vi "Weather Parse Test.vi"() -> ()   [LabVIEW 2020, in "CDM-Config.lvlib"] (continued)
MI and Port Austin to Harbor Beach MI.\\n\\n* WHEN...The maximum winds are expected around 7 AM EST Thursday\\nwith the largest waves expected around 9 AM EST Thursday.\\n\\n* IMPACTS...Conditions will be hazardous to small craft.\",\n                \"instruction\": \"Inexperienced mariners, especially those operating smaller\\nvessels, should avoid navigating in hazardous conditions.\",\n                \"response\": \"Avoid\",\n                \"parameters\": {\n                    \"AWIPSidentifier\": [\n                        \"MWWDTX\"\n                    ],\n                    \"WMOidentifier\": [\n                        \"WHUS73 KDTX 030901\"\n                    ],\n                    \"NWSheadline\": [\n                        \"SMALL CRAFT ADVISORY REMAINS IN EFFECT UNTIL 4 PM EST THURSDAY\"\n                    ],\n                    \"BLOCKCHANNEL\": [\n                        \"EAS\",\n                        \"NWEM\",\n                        \"CMAS\"\n                    ],\n                    \"VTEC\": [\n                        \"/O.CON.KDTX.SC.Y.0091.000000T0000Z-251204T2100Z/\"\n                    ],\n                    \"eventEndingTime\": [\n                        \"2025-12-04T16:00:00-05:00\"\n                    ],\n                    \"expiredReferences\": [\n                        \"w-nws.webmaster@noaa.gov,urn:oid:2.49.0.1.840.0.2ff8cea4919408243d7957368d495bee02ffd6db.001.1,2025-12-02T03:07:00-05:00\"\n                    ]\n                },\n                \"scope\": \"Public\",\n                \"code\": \"IPAWSv1.0\",\n                \"language\": \"en-US\",\n                \"web\": \"http://www.weather.gov\",\n                \"eventCode\": {\n                    \"SAME\": [\n                        \"NWS\"\n                    ],\n                    \"NationalWeatherService\": [\n                        \"SCY\"\n                    ]\n                }\n            }\n        },\n        {\n            \"id\": \"https://api.weather.gov/alerts/urn:oid:2.49.0.1.840.0.dab1393c914b230290374bee41bf50b08330d8fe.001.1\",\n            \"type\": \"Feature\",\n            \"geometry\": null,\n            \"properties\": {\n                \"@id\": \"https://api.weather.gov/alerts/urn:oid:2.49.0.1.840.0.dab1393c914b230290374bee41bf50b08330d8fe.001.1\",\n                \"@type\": \"wx:Alert\",\n                \"id\": \"urn:oid:2.49.0.1.840.0.dab1393c914b230290374bee41bf50b08330d8fe.001.1\",\n                \"areaDesc\": \"Harbor Beach to Port Sanilac MI; Port Sanilac to Port Huron MI\",\n                \"geocode\": {\n                    \"SAME\": [\n                        \"093442\",\n                        \"093443\"\n                    ],\n                    \"UGC\": [\n                        \"LHZ442\",\n                        \"LHZ443\"\n                    ]\n                },\n                \"affectedZones\": [\n                    \"https://api.weather.gov/zones/forecast/LHZ442\",\n                    \"https://api.weather.gov/zones/forecast/LHZ443\"\n                ],\n                \"references\": [],\n                \"sent\": \"2025-12-03T04:01:00-05:00\",\n                \"effective\": \"2025-12-03T04:01:00-05:00\",\n                \"onset\": \"2025-12-03T22:00:00-05:00\",\n                \"expires\": \"2025-12-03T16:15:00-05:00\",\n                \"ends\": \"2025-12-04T16:00:00-05:00\",\n                \"status\": \"Actual\",\n                \"messageType\": \"Alert\",\n                \"category\": \"Met\",\n                \"severity\": \"Minor\",\n                \"certainty\": \"Likely\",\n                \"urgency\": \"Expected\",\n                \"event\": \"Small Craft Advisory\",\n                \"sender\": \"w-nws.webmaster@noaa.gov\",\n                \"senderName\": \"NWS Detroit/Pontiac MI\",\n                \"headline\": \"Small Craft Advisory issued December 3 at 4:01AM EST until December 4 at 4:00PM EST by NWS Detroit/Pontiac MI\",\n                \"description\": \"* WHAT...Expect sustained winds up to 23 knots from the northwest\\nwith gusts up to 30 knots. The largest significant waves will\\nbe 4 feet with a potential maximum wave height of 5 feet.\\n\\n* WHERE...Harbor Beach to Port Sanilac MI and Port Sanilac to\\nPort Huron MI.\\n\\n* WHEN...The maximum winds are expected around 6 AM EST Thursday\\nwith the largest waves expected around 9 AM EST Thursday.\\n\\n* IMPACTS...Conditions will be hazardous to small craft.\",\n                \"instruction\": \"Inexperienced mariners, especially those operating smaller\\nvessels, should avoid navigating in hazardous conditions.\",\n                \"response\": \"Avoid\",\n                \"parameters\": {\n                    \"AWIPSidentifier\": [\n                        \"MWWDTX\"\n                    ],\n                    \"WMOidentifier\": [\n                        \"WHUS73 KDTX 030901\"\n                    ],\n                    \"NWSheadline\": [\n                        \"SMALL CRAFT ADVISORY IN EFFECT FROM 10 PM THIS EVENING TO 4 PM EST THURSDAY\"\n                    ],\n                    \"BLOCKCHANNEL\": [\n                        \"EAS\",\n                        \"NWEM\",\n                        \"CMAS\"\n                    ],\n                    \"VTEC\": [\n                        \"/O.EXB.KDTX.SC.Y.0091.251204T0300Z-251204T2100Z/\"\n                    ],\n                    \"eventEndingTime\": [\n                        \"2025-12-04T16:00:00-05:00\"\n                    ]\n                },\n                \"scope\": \"Public\",\n                \"code\": \"IPAWSv1.0\",\n                \"language\": \"en-US\",\n                \"web\": \"http://www.weather.gov\",\n                \"eventCode\": {\n                    \"SAME\": [\n                        \"NWS\"\n                    ],\n                    \"NationalWeatherService\": [\n                        \"SCY\"\n                    ]\n                }\n            }\n        },\n        {\n            \"id\": \"https://api.weather.gov/alerts/urn:oid:2.49.0.1.840.0.0ce6f9fefeeb8151c750e6368d77a21669e0c8b3.001.1\",\n            \"type\": \"Feature\",\n            \"geometry\": null,\n            \"properties\": {\n                \"@id\": \"https://api.weather.gov/alerts/urn:oid:2.49.0.1.840.0.0ce6f9fefeeb8151c750e6368d77a21669e0c8b3.001.1\",\n                \"@type\": \"wx:Alert\",\n                \"id\": \"urn:oid:2.49.0.1.840.0.0ce6f9fefeeb8151c750e6368d77a21669e0c8b3.001.1\",\n                \"areaDesc\": \"Lake Mead National Recreation Area; Lake Mead National Recreation Area\",\n                \"geocode\": {\n                    \"SAME\": [\n                        \"004015\",\n                        \"032003\"\n                    ],\n                    \"UGC\": [\n                        \"AZZ036\",\n                        \"NVZ021\"\n                    ]\n                },\n                \"affectedZones\": [\n                    \"https://api.weather.gov/zones/forecast/AZZ036\",\n                    \"https://api.weather.gov/zones/forecast/NVZ021\"\n                ],\n                \"references\": [\n                    {\n                        \"@id\": \"https://api.weather.gov/alerts/urn:oid:2.49.0.1.840.0.e1ccc9c98ec3a9bf71d0b8eee838f53e2100c777.001.1\",\n                        \"identifier\": \"urn:oid:2.49.0.1.840.0.e1ccc9c98ec3a9bf71d0b8eee838f53e2100c777.001.1\",\n                        \"sender\": \"w-nws.webmaster@noaa.gov\",\n                        \"sent\": \"2025-12-02T10:39:00-08:00\"\n                    }\n                ],\n                \"sent\": \"2025-12-03T00:46:00-08:00\",\n                \"effective\": \"2025-12-03T00:46:00-08:00\",\n                \"onset\": \"2025-12-03T09:00:00-08:00\",\n                \"expires\": \"2025-12-03T18:00:00-08:00\",\n                \"ends\": \"2025-12-03T18:00:00-08:00\",\n                \"status\": \"Actual\",\n                \"messageType\": \"Update\",\n                \"category\": \"Met\",\n                \"severity\": \"Moderate\",\n                \"certainty\": \"Likely\",\n                \"urgency\": \"Expected\",\n                \"event\": \"Lake Wind Advisory\",\n                \"sender\": \"w-nws.webmaster@noaa.gov\",\n                \"senderName\": \"NWS Las Vegas NV\",\n                \"headline\": \"Lake Wind Advisory issued December 3 at 12:46AM PST until December 3 at 6:00PM PST by NWS Las Vegas NV\",\n                \"description\": \"* WHAT...North winds 15 to 25 mph with gusts up to 35 mph expected.\\nWave heights 2 to 3 feet on Lake Mohave.\\n\\n* WHERE...Lake Mead and Lake Mohave.\\n\\n* WHEN...From 9 AM PST /10 AM MST/ this morning to 6 PM PST /7 PM\\nMST/ this evening.\\n\\n* IMPACTS...Strong winds and rough waves on area lakes will create\\nhazardous conditions for small craft.\",\n                \"instruction\": \"Winds this strong can make driving difficult, especially for high\\nprofile vehicles. Use extra caution.\",\n                \"response\": \"Execute\",\n                \"parameters\": {\n                    \"AWIPSidentifier\": [\n                        \"NPWVEF\"\n                    ],\n                    \"WMOidentifier\": [\n                        \"WWUS75 KVEF 030846\"\n                    ],\n                    \"NWSheadline\": [\n                        \"LAKE WIND ADVISORY REMAINS IN EFFECT FROM 9 AM PST /10 AM MST/ THIS MORNING TO 6 PM PST /7 PM MST/ THIS EVENING\"\n                    ],\n                    \"BLOCKCHANNEL\": [\n                        \"EAS\",\n                        \"NWEM\",\n                        \"CMAS\"\n                    ],\n                    \"VTEC\": [\n                        \"/O.CON.KVEF.LW.Y.0010.251203T1700Z-251204T0200Z/\"\n                    ],\n                    \"eventEndingTime\": [\n                        \"2025-12-03T18:00:00-08:00\"\n                    ]\n                },\n                \"scope\": \"Public\",\n                \"code\": \"IPAWSv1.0\",\n                \"language\": \"en-US\",\n                \"web\": \"http://www.weather.gov\",\n                \"eventCode\": {\n                    \"SAME\": [\n                        \"NWS\"\n                    ],\n                    \"NationalWeatherService\": [\n                        \"LWY\"\n                    ]\n                }\n            }\n        },\n        {\n            \"id\": \"https://api.weather.gov/alerts/urn:oid:2.49.0.1.840.0.0594a10134f977bf8f2849286ea6b737812d75ba.001.2\",\n            \"type\": \"Feature\",\n            \"geometry\": null,\n            \"properties\": {\n                \"@id\": \"https://api.weather.gov/alerts/urn:oid:2.49.0.1.840.0.0594a10134f977bf8f2849286ea6b737812d75ba.001.2\",\n                \"@type\": \"wx:Alert\",\n                \"id\": \"urn:oid:2.49.0.1.840.0.0594a10134f977bf8f2849286ea6b737812d75ba.001.2\",\n                \"areaDesc\": \"Northern Sangre de Cristo Mountains; East Slopes Sangre de Cristo Mountains; Johnson and Bartlett Mesas Including Raton Pass\",\n                \"geocode\": {\n                    \"SAME\": [\n                        \"035007\",\n                        \"035055\",\n                        \"035033\",\n                        \"035047\",\n                        \"035059\"\n                    ],\n                    \"UGC\": [\n                        \"NMZ213\",\n                        \"NMZ215\",\n                        \"NMZ227\"\n                    ]\n                },\n                \"affectedZones\": [\n                    \"https://api.weather.gov/zones/forecast/NMZ213\",\n                    \"https://api.weather.gov/zones/forecast/NMZ215\",\n                    \"https://api.weather.gov/zones/forecast/NMZ227\"\n                ],\n                \"references\": [],\n                \"sent\": \"2025-12-03T01:43:00-07:00\",\n                \"effective\": \"2025-12-03T01:43:00-07:00\",\n                \"onset\": \"2025-12-03T12:00:00-07:00\",\n                \"expires\": \"2025-12-03T12:00:00-07:00\",\n                \"ends\": \"2025-12-04T05:00:00-07:00\",\n                \"status\": \"Actual\",\n                \"messageType\": \"Alert\",\n                \"category\": \"Met\",\n                \"severity\": \"Severe\",\n                \"certainty\": \"Likely\",\n                \"urgency\": \"Expected\",\n                \"event\": \"Winter Storm Warning\",\n                \"sender\": \"w-nws.webmaster@noaa.gov\",\n                \"senderName\": \"NWS Albuquerque NM\",\n                \"headline\": \"Winter Storm Warning issued December 3 at 1:43AM MST until December 4 at 5:00AM MST by NWS Albuquerque NM\",\n                \"description\": \"* WHAT...Heavy snow expected. Total snow accumulations between 6 and\\n12 inches, except up to 15 inches in the mountains near the\\nColorado border, and 3 to 6 inches below 7500 feet.\\n\\n* WHERE...East Slopes Sangre de Cristo Mountains, Northern Sangre de\\nCristo Mountains, and Johnson and Bartlett Mesas Including Raton\\nPass.\\n\\n* WHEN...From noon today to 5 AM MST Thursday.\\n\\n* IMPACTS...Travel could be very difficult. Tire traction will be\\nreduced. Extend the distance between your vehicle and the vehicle\\nin front of you. This includes I-25 over Raton Pass. The hazardous\\nconditions will impact commutes this evening and Thursday morning.\\n\\n* ADDITIONAL DETAILS...Snow will begin to accumulate near the\\nColorado border late this morning, then accumulating snow will\\nbecome widespread in the afternoon. The heaviest snowfall is\\nexpected this evening, when the visibility will drop below a\\nquarter mile at times.\",\n                \"instruction\": \"If you must travel, keep an extra flashlight, food, and water in\\nyour vehicle in case of an emergency. For the latest road\\nconditions, dial 511 or 1.800.432.4269, or visit http://nmroads.com.\",\n                \"response\": \"Prepare\",\n                \"parameters\": {\n                    \"AWIPSidentifier\": [\n                        \"WSWABQ\"\n                    ],\n                    \"WMOidentifier\": [\n                        \"WWUS45 KABQ 030843\"\n                    ],\n                    \"NWSheadline\": [\n                        \"WINTER STORM WARNING IN EFFECT FROM NOON TODAY TO 5 AM MST THURSDAY\"\n                    ],\n                    \"BLOCKCHANNEL\": [\n                        \"EAS\",\n                        \"NWEM\",\n                        \"CMAS\"\n                    ],\n                    \"EAS-ORG\": [\n                        \"WXR\"\n                    ],\n                    \"VTEC\": [\n                        \"/O.NEW.KABQ.WS.W.0010.251203T1900Z-251204T1200Z/\"\n                    ],\n                    \"eventEndingTime\": [\n                        \"2025-12-04T05:00:00-07:00\"\n                    ]\n                },\n                \"scope\": \"Public\",\n                \"code\": \"IPAWSv1.0\",\n                \"language\": \"en-US\",\n                \"web\": \"http://www.weather.gov\",\n                \"eventCode\": {\n                    \"SAME\": [\n                        \"WSW\"\n                    ],\n                    \"NationalWeatherService\": [\n                        \"WSW\"\n                    ]\n                }\n            }\n        },\n        {\n            \"id\": \"https://api.weather.gov/alerts/urn:oid:2.49.0.1.840.0.0594a10134f977bf8f2849286ea6b737812d75ba.005.1\",\n            \"type\": \"Feature\",\n            \"geometry\": null,\n            \"properties\": {\n                \"@id\": \"https://api.weather.gov/alerts/urn:oid:2.49.0.1.840.0.0594a10134f977bf8f2849286ea6b737812d75ba.005.1\",\n                \"@type\": \"wx:Alert\",\n                \"id\": \"urn:oid:2.49.0.1.840.0.0594a10134f977bf8f2849286ea6b737812d75ba.005.1\",\n                \"areaDesc\": \"Central Highlands\",\n                \"geocode\": {\n                    \"SAME\": [\n                        \"035047\",\n                        \"035049\",\n                        \"035057\"\n                    ],\n                    \"UGC\": [\n                        \"NMZ223\"\n                    ]\n                },\n                \"affectedZones\": [\n                    \"https://api.weather.gov/zones/forecast/NMZ223\"\n                ],\n                \"references\": [\n                    {\n                        \"@id\": \"https://api.weather.gov/alerts/urn:oid:2.49.0.1.840.0.941388ae9bb36314f84811b9b5bde722294ef589.002.1\",\n                        \"identifier\": \"urn:oid:2.49.0.1.840.0.941388ae9bb36314f84811b9b5bde722294ef589.002.1\",\n                        \"sender\": \"w-nws.webmaster@noaa.gov\",\n                        \"sent\": \"2025-12-02T18:02:00-07:00\"\n                    }\n                ],\n                \"sent\": \"2025-12-03T01:43:00-07:00\",\n                \"effective\": \"2025-12-03T01:43:00-07:00\",\n                \"onset\": \"2025-12-03T17:00:00-07:00\",\n                \"expires\": \"2025-12-03T12:00:00-07:00\",\n                \"ends\": \"2025-12-04T05:00:00-07:00\",\n                \"status\": \"Actual\",\n                \"messageType\": \"Update\",\n                \"category\": \"Met\",\n                \"severity\": \"Moderate\",\n                \"certainty\": \"Likely\",\n                \"urgency\": \"Expected\",\n                \"event\": \"Winter Weather Advisory\",\n                \"sender\": \"w-nws.webmaster@noaa.gov\",\n                \"senderName\": \"NWS Albuquerque NM\",\n                \"headline\": \"Winter Weather Advisory issued December 3 at 1:43AM MST until December 4 at 5:00AM MST by NWS Albuquerque NM\",\n                \"description\": \"* WHAT...Snow expected. Total snow accumulations between 1 and 4\\ninches.\\n\\n* WHERE...Central Highlands.\\n\\n* WHEN...From 5 PM this afternoon to 5 AM MST Thursday.\\n\\n* IMPACTS...Plan on snow packed or icy road conditions for commutes\\nthis evening and Thursday morning. This includes I-40 between\\nMoriarty and Santa Rosa, including Clines Corners.\\n\\n* ADDITIONAL DETAILS...The heaviest snowfall will occur this evening\\nwhen the visibility will drop below a half mile at times.\",\n                \"instruction\": \"Slow down and use caution while traveling. For the latest road\\nconditions, dial 511 or 1.800.432.4269, or visit http://nmroads.com.\",\n                \"response\": \"Execute\",\n                \"parameters\": {\n                    \"AWIPSidentifier\": [\n                        \"WSWABQ\"\n                    ],\n                    \"WMOidentifier\": [\n                        \"WWUS45 KABQ 030843\"\n                    ],\n                    \"NWSheadline\": [\n                        \"WINTER WEATHER ADVISORY REMAINS IN EFFECT FROM 5 PM THIS AFTERNOON TO 5 AM MST THURSDAY\"\n                    ],\n                    \"BLOCKCHANNEL\": [\n                        \"EAS\",\n                        \"NWEM\",\n                        \"CMAS\"\n                    ],\n                    \"VTEC\": [\n                        \"/O.CON.KABQ.WW.Y.0019.251204T0000Z-251204T1200Z/\"\n                    ],\n                    \"eventEndingTime\": [\n                        \"2025-12-04T05:00:00-07:00\"\n                    ],\n                    \"expiredReferences\": [\n                        \"w-nws.webmaster@noaa.gov,urn:oid:2.49.0.1.840.0.c3d145e831a7a2c0d935c1490f6242d68170c4ec.002.1,2025-12-02T09:55:00-07:00\"\n                    ]\n                },\n                \"scope\": \"Public\",\n                \"code\": \"IPAWSv1.0\",\n                \"language\": \"en-US\",\n                \"web\": \"http://www.weather.gov\",\n                \"eventCode\": {\n                    \"SAME\": [\n                        \"NWS\"\n                    ],\n                    \"NationalWeatherService\": [\n                        \"WWY\"\n                    ]\n                }\n            }\n        },\n        {\n            \"id\": \"https://api.weather.gov/alerts/urn:oid:2.49.0.1.840.0.0594a10134f977bf8f2849286ea6b737812d75ba.003.1\",\n            \"type\": \"Feature\",\n            \"geometry\": null,\n            \"properties\": {\n                \"@id\": \"https://api.weather.gov/alerts/urn:oid:2.49.0.1.840.0.0594a10134f977bf8f2849286ea6b737812d75ba.003.1\",\n                \"@type\": \"wx:Alert\",\n                \"id\": \"urn:oid:2.49.0.1.840.0.0594a10134f977bf8f2849286ea6b737812d75ba.003.1\",\n                \"areaDesc\": \"Sandia/Manzano Mountains Including Edgewood\",\n                \"geocode\": {\n                    \"SAME\": [\n                        \"035001\",\n                        \"035043\",\n                        \"035049\",\n                        \"035057\",\n                        \"035061\"\n                    ],\n                    \"UGC\": [\n                        \"NMZ221\"\n                    ]\n                },\n                \"affectedZones\": [\n                    \"https://api.weather.gov/zones/forecast/NMZ221\"\n                ],\n                \"references\": [],\n                \"sent\": \"2025-12-03T01:43:00-07:00\",\n                \"effective\": \"2025-12-03T01:43:00-07:00\",\n                \"onset\": \"2025-12-03T17:00:00-07:00\",\n                \"expires\": \"2025-12-03T12:00:00-07:00\",\n                \"ends\": \"2025-12-04T05:00:00-07:00\",\n                \"status\": \"Actual\",\n                \"messageType\": \"Alert\",\n                \"category\": \"Met\",\n                \"severity\": \"Moderate\",\n                \"certainty\": \"Likely\",\n                \"urgency\": \"Expected\",\n                \"event\": \"Winter Weather Advisory\",\n                \"sender\": \"w-nws.webmaster@noaa.gov\",\n                \"senderName\": \"NWS Albuquerque NM\",\n                \"headline\": \"Winter Weather Advisory issued December 3 at 1:43AM MST until December 4 at 5:00AM MST by NWS Albuquerque NM\",\n                \"description\": \"* WHAT...Snow expected. Total snow accumulations between 2 and 5\\ninches, with locally higher amounts on Sandia Crest.\\n\\n* WHERE...Sandia and Manzano Mountains including Edgewood.\\n\\n* WHEN...From 5 PM this afternoon to 5 AM MST Thursday.\\n\\n* IMPACTS...Plan on snow packed or icy road conditions for commutes\\nthis evening and Thursday morning. This includes I-40 through\\nTijeras Canyon.\\n\\n* ADDITIONAL DETAILS...The heaviest snow will occur this evening,\\nwhen the visibility will drop below a quarter mile at times in\\nblowing snow. East canyon wind gusts up to 35 mph during the\\nevening and through the late night hours.\",\n                \"instruction\": \"Slow down and use caution while traveling. For the latest road\\nconditions, dial 511 or 1.800.432.4269, or visit http://nmroads.com.\",\n                \"response\": \"Execute\",\n                \"parameters\": {\n                    \"AWIPSidentifier\": [\n                        \"WSWABQ\"\n                    ],\n                    \"WMOidentifier\": [\n                        \"WWUS45 KABQ 030843\"\n                    ],\n                    \"NWSheadline\": [\n                        \"WINTER WEATHER ADVISORY IN EFFECT FROM 5 PM THIS AFTERNOON TO 5 AM MST THURSDAY\"\n                    ],\n                    \"BLOCKCHANNEL\": [\n                        \"EAS\",\n                        \"NWEM\",\n                        \"CMAS\"\n                    ],\n                    \"VTEC\": [\n                        \"/O.EXA.KABQ.WW.Y.0019.251204T0000Z-251204T1200Z/\"\n                    ],\n                    \"eventEndingTime\": [\n                        \"2025-12-04T05:00:00-07:00\"\n                    ]\n                },\n                \"scope\": \"Public\",\n                \"code\": \"IPAWSv1.0\",\n                \"language\": \"en-US\",\n                \"web\": \"http://www.weather.gov\",\n                \"eventCode\": {\n                    \"SAME\": [\n                        \"NWS\"\n                    ],\n                    \"NationalWeatherService\": [\n                        \"WWY\"\n                    ]\n                }\n            }\n        },\n        {\n            \"id\": \"https://api.weather.gov/alerts/urn:oid:2.49.0.1.840.0.0594a10134f977bf8f2849286ea6b737812d75ba.002.1\",\n            \"type\": \"Feature\",\n            \"geometry\": null,\n            \"properties\": {\n                \"@id\": \"https://api.weather.gov/alerts/urn:oid:2.49.0.1.840.0.0594a10134f977bf8f2849286ea6b737812d75ba.002.1\",\n                \"@type\": \"wx:Alert\",\n                \"id\": \"urn:oid:2.49.0.1.840.0.0594a10134f977bf8f2849286ea6b737812d75ba.002.1\",\n                \"areaDesc\": \"Far Northwest Highlands; Jemez Mountains\",\n                \"geocode\": {\n                    \"SAME\": [\n                        \"035039\",\n                        \"035043\",\n                        \"035045\",\n                        \"035028\"\n                    ],\n                    \"UGC\": [\n                        \"NMZ203\",\n                        \"NMZ211\"\n                    ]\n                },\n                \"affectedZones\": [\n                    \"https://api.weather.gov/zones/forecast/NMZ203\",\n                    \"https://api.weather.gov/zones/forecast/NMZ211\"\n                ],\n                \"references\": [],\n                \"sent\": \"2025-12-03T01:43:00-07:00\",\n                \"effective\": \"2025-12-03T01:43:00-07:00\",\n                \"onset\": \"2025-12-03T12:00:00-07:00\",\n                \"expires\": \"2025-12-03T12:00:00-07:00\",\n                \"ends\": \"2025-12-04T05:00:00-07:00\",\n                \"status\": \"Actual\",\n                \"messageType\": \"Alert\",\n                \"category\": \"Met\",\n                \"severity\": \"Moderate\",\n                \"certainty\": \"Likely\",\n                \"urgency\": \"Expected\",\n                \"event\": \"Winter Weather Advisory\",\n                \"sender\": \"w-nws.webmaster@noaa.gov\",\n                \"senderName\": \"NWS Albuquerque NM\",\n                \"headline\": \"Winter Weather Advisory issued December 3 at 1:43AM MST until December 4 at 5:00AM MST by NWS Albuquerque NM\",\n                \"description\": \"* WHAT...Snow expected. Total snow accumulations between 1 and 3\\ninches, except 3 to 6 inches above 7500 feet.  Locally higher\\namounts near 8 inches along the east slopes of the Jemez Mountains.\\n\\n* WHERE...Far Northwest Highlands and Jemez Mountains.\\n\\n* WHEN...From noon today to 5 AM MST Thursday.\\n\\n* IMPACTS...Plan on snow packed or icy road conditions. The\\nhazardous conditions will impact commutes this evening and\\nThursday morning.\\n\\n* ADDITIONAL DETAILS...Snow will begin to accumulate near the\\nColorado border late this morning, then accumulating snow will\\nspread to the Jemez Mountains as well during the afternoon. The\\nheaviest snowfall will occur Wednesday evening in most places,\\nwhen the visibility will drop below a half mile at times.\",\n                \"instruction\": \"Slow down and use caution while traveling. For the latest road\\nconditions, dial 511 or 1.800.432.4269, or visit http://nmroads.com.\",\n                \"response\": \"Execute\",\n                \"parameters\": {\n                    \"AWIPSidentifier\": [\n                        \"WSWABQ\"\n                    ],\n                    \"WMOidentifier\": [\n                        \"WWUS45 KABQ 030843\"\n                    ],\n                    \"NWSheadline\": [\n                        \"WINTER WEATHER ADVISORY IN EFFECT FROM NOON TODAY TO 5 AM MST THURSDAY\"\n                    ],\n                    \"BLOCKCHANNEL\": [\n                        \"EAS\",\n                        \"NWEM\",\n                        \"CMAS\"\n                    ],\n                    \"VTEC\": [\n                        \"/O.EXA.KABQ.WW.Y.0019.251203T1900Z-251204T1200Z/\"\n                    ],\n                    \"eventEndingTime\": [\n                        \"2025-12-04T05:00:00-07:00\"\n                    ]\n                },\n                \"scope\": \"Public\",\n                \"code\": \"IPAWSv1.0\",\n                \"language\": \"en-US\",\n                \"web\": \"http://www.weather.gov\",\n                \"eventCode\": {\n                    \"SAME\": [\n                        \"NWS\"\n                    ],\n                    \"NationalWeatherService\": [\n                        \"WWY\"\n                    ]\n                }\n            }\n        },\n        {\n            \"id\": \"https://api.weather.gov/alerts/urn:oid:2.49.0.1.840.0.0594a10134f977bf8f2849286ea6b737812d75ba.004.1\",\n            \"type\": \"Feature\",\n            \"geometry\": null,\n            \"properties\": {\n                \"@id\": \"https://api.weather.gov/alerts/urn:oid:2.49.0.1.840.0.0594a10134f977bf8f2849286ea6b737812d75ba.004.1\",\n                \"@type\": \"wx:Alert\",\n                \"id\": \"urn:oid:2.49.0.1.840.0.0594a10134f977bf8f2849286ea6b737812d75ba.004.1\",\n                \"areaDesc\": \"Tusas Mountains Including Chama; Glorieta Mesa Including Glorieta Pass; Southern Sangre de Cristo Mountains; Upper Rio Grande Valley; Far Northeast Highlands; Northeast Highlands\",\n                \"geocode\": {\n                    \"SAME\": [\n                        \"035039\",\n                        \"035055\",\n                        \"035047\",\n                        \"035049\",\n                        \"035007\",\n                        \"035033\"\n                    ],\n                    \"UGC\": [\n                        \"NMZ210\",\n                        \"NMZ212\",\n                        \"NMZ214\",\n                        \"NMZ216\",\n                        \"NMZ228\",\n                        \"NMZ229\"\n                    ]\n                },\n                \"affectedZones\": [\n                    \"https://api.weather.gov/zones/forecast/NMZ210\",\n                    \"https://api.weather.gov/zones/forecast/NMZ212\",\n                    \"https://api.weather.gov/zones/forecast/NMZ214\",\n                    \"https://api.weather.gov/zones/forecast/NMZ216\",\n                    \"https://api.weather.gov/zones/forecast/NMZ228\",\n                    \"https://api.weather.gov/zones/forecast/NMZ229\"\n                ],\n                \"references\": [\n                    {\n                        \"@id\": \"https://api.weather.gov/alerts/urn:oid:2.49.0.1.840.0.941388ae9bb36314f84811b9b5bde722294ef589.001.1\",\n                        \"identifier\": \"urn:oid:2.49.0.1.840.0.941388ae9bb36314f84811b9b5bde722294ef589.001.1\",\n                        \"sender\": \"w-nws.webmaster@noaa.gov\",\n                        \"sent\": \"2025-12-02T18:02:00-07:00\"\n                    }\n                ],\n                \"sent\": \"2025-12-03T01:43:00-07:00\",\n                \"effective\": \"2025-12-03T01:43:00-07:00\",\n                \"onset\": \"2025-12-03T12:00:00-07:00\",\n                \"expires\": \"2025-12-03T12:00:00-07:00\",\n                \"ends\": \"2025-12-04T05:00:00-07:00\",\n                \"status\": \"Actual\",\n                \"messageType\": \"Update\",\n                \"category\": \"Met\",\n                \"severity\": \"Moderate\",\n                \"certainty\": \"Likely\",\n                \"urgency\": \"Expected\",\n                \"event\": \"Winter Weather Advisory\",\n                \"sender\": \"w-nws.webmaster@noaa.gov\",\n                \"senderName\": \"NWS Albuquerque NM\",\n                \"headline\": \"Winter Weather Advisory issued December 3 at 1:43AM MST until December 4 at 5:00AM MST by NWS Albuquerque NM\",\n                \"description\": \"* WHAT...Snow expected. Total snow accumulations between 1 and 4\\ninches below 7500 feet, and between 4 and 8 inches above 7500\\nfeet. Locally up to 10 inches on the highest peaks of the Sangre\\nde Cristo Mountains.\\n\\n* WHERE...Glorieta Mesa Including Glorieta Pass, Southern Sangre de\\nCristo Mountains, Tusas Mountains Including Chama, Upper Rio\\nGrande Valley, Far Northeast Highlands, and Northeast Highlands.\\n\\n* WHEN...From noon today to 5 AM MST Thursday.\\n\\n* IMPACTS...Travel could be very difficult. Tire traction will be\\nreduced. Extend the distance between your vehicle and the vehicle\\nin front of you. This includes I-25 over Glorieta Pass. The\\nhazardous conditions will impact commutes this evening and\\nThursday morning.\\n\\n* ADDITIONAL DETAILS...Snow will begin to accumulate near the\\nColorado border this morning, then spread further south this\\nafternoon.  The heaviest snowfall in most locations will occur\\nthis evening when the visibility will drop below a half mile at\\ntimes.\",\n                \"instruction\": \"Slow down and use caution while traveling. For the latest road\\nconditions, dial 511 or 1.800.432.4269, or visit http://nmroads.com.\",\n                \"response\": \"Execute\",\n                \"parameters\": {\n                    \"AWIPSidentifier\": [\n                        \"WSWABQ\"\n                    ],\n                    \"WMOidentifier\": [\n                        \"WWUS45 KABQ 030843\"\n                    ],\n                    \"NWSheadline\": [\n                        \"WINTER WEATHER ADVISORY REMAINS IN EFFECT FROM NOON TODAY TO 5 AM MST THURSDAY\"\n                    ],\n                    \"BLOCKCHANNEL\": [\n                        \"EAS\",\n                        \"NWEM\",\n                        \"CMAS\"\n                    ],\n                    \"VTEC\": [\n                        \"/O.CON.KABQ.WW.Y.0019.251203T1900Z-251204T1200Z/\"\n                    ],\n                    \"eventEndingTime\": [\n                        \"2025-12-04T05:00:00-07:00\"\n                    ],\n                    \"expiredReferences\": [\n                        \"w-nws.webmaster@noaa.gov,urn:oid:2.49.0.1.840.0.c3d145e831a7a2c0d935c1490f6242d68170c4ec.003.1,2025-12-02T09:55:00-07:00 w-nws.webmaster@noaa.gov,urn:oid:2.49.0.1.840.0.c3d145e831a7a2c0d935c1490f6242d68170c4ec.001.1,2025-12-02T09:55:00-07:00 w-nws.webmaster@noaa.gov,urn:oid:2.49.0.1.840.0.0ace8003fd2e1ec30d59fe0304cfb7a59138cfec.001.1,2025-12-02T02:40:00-07:00\"\n                    ]\n                },\n                \"scope\": \"Public\",\n                \"code\": \"IPAWSv1.0\",\n                \"language\": \"en-US\",\n                \"web\": \"http://www.weather.gov\",\n                \"eventCode\": {\n                    \"SAME\": [\n                        \"NWS\"\n                    ],\n                    \"NationalWeatherService\": [\n                        \"WWY\"\n                    ]\n                }\n            }\n        },\n        {\n            \"id\": \"https://api.weather.gov/alerts/urn:oid:2.49.0.1.840.0.810f735991b3c019dc43a3db04dbca83dd500741.001.1\",\n            \"type\": \"Feature\",\n            \"geometry\": null,\n            \"properties\": {\n                \"@id\": \"https://api.weather.gov/alerts/urn:oid:2.49.0.1.840.0.810f735991b3c019dc43a3db04dbca83dd500741.001.1\",\n                \"@type\": \"wx:Alert\",\n                \"id\": \"urn:oid:2.49.0.1.840.0.810f735991b3c019dc43a3db04dbca83dd500741.001.1\",\n                \"areaDesc\": \"Greater Lake Tahoe Area; Greater Lake Tahoe Area\",\n                \"geocode\": {\n                    \"SAME\": [\n                        \"006003\",\n                        \"006017\",\n                        \"006057\",\n                        \"006061\",\n                        \"032005\",\n                        \"032031\",\n                        \"032510\"\n                    ],\n                    \"UGC\": [\n                        \"CAZ072\",\n                        \"NVZ002\"\n                    ]\n                },\n                \"affectedZones\": [\n                    \"https://api.weather.gov/zones/forecast/CAZ072\",\n                    \"https://api.weather.gov/zones/forecast/NVZ002\"\n                ],\n                \"references\": [],\n                \"sent\": \"2025-12-03T00:34:00-08:00\",\n                \"effective\": \"2025-12-03T00:34:00-08:00\",\n                \"onset\": \"2025-12-03T00:34:00-08:00\",\n                \"expires\": \"2025-12-03T10:00:00-08:00\",\n                \"ends\": \"2025-12-03T10:00:00-08:00\",\n                \"status\": \"Actual\",\n                \"messageType\": \"Alert\",\n                \"category\": \"Met\",\n                \"severity\": \"Moderate\",\n                \"certainty\": \"Likely\",\n                \"urgency\": \"Expected\",\n                \"event\": \"Lake Wind Advisory\",\n                \"sender\": \"w-nws.webmaster@noaa.gov\",\n                \"senderName\": \"NWS Reno NV\",\n                \"headline\": \"Lake Wind Advisory issued December 3 at 12:34AM PST until December 3 at 10:00AM PST by NWS Reno NV\",\n                \"description\": \"* WHAT...East winds 15 to 20 mph with gusts up to 35 mph and waves 1\\nto 3 feet for Lake Tahoe.\\n\\n* WHERE...Greater Lake Tahoe Area.\\n\\n* WHEN...Until 10 AM PST this morning.\\n\\n* IMPACTS...Small boats, kayaks and paddle boards will be prone to\\ncapsizing and should remain off lake waters until conditions\\nimprove.\\n\\n* ADDITIONAL DETAILS...The strongest winds and highest waves will\\noccur over the southwest portion of Lake Tahoe.\",\n                \"instruction\": \"Check lake conditions before heading out and be prepared for a\\nsudden increase in winds and wave heights. Consider postponing\\nboating activities on the lake until a day with less wind.\",\n                \"response\": \"Execute\",\n                \"parameters\": {\n                    \"AWIPSidentifier\": [\n                        \"NPWREV\"\n                    ],\n                    \"WMOidentifier\": [\n                        \"WWUS75 KREV 030834\"\n                    ],\n                    \"NWSheadline\": [\n                        \"LAKE WIND ADVISORY IN EFFECT UNTIL 10 AM PST THIS MORNING FOR LAKE TAHOE\"\n                    ],\n                    \"BLOCKCHANNEL\": [\n                        \"EAS\",\n                        \"NWEM\",\n                        \"CMAS\"\n                    ],\n                    \"VTEC\": [\n                        \"/O.NEW.KREV.LW.Y.0041.251203T0834Z-251203T1800Z/\"\n                    ],\n                    \"eventEndingTime\": [\n                        \"2025-12-03T10:00:00-08:00\"\n                    ]\n                },\n                \"scope\": \"Public\",\n                \"code\": \"IPAWSv1.0\",\n                \"language\": \"en-US\",\n                \"web\": \"http://www.weather.gov\",\n                \"eventCode\": {\n                    \"SAME\": [\n                        \"NWS\"\n                    ],\n                    \"NationalWeatherService\": [\n                        \"LWY\"\n                    ]\n                }\n            }\n        },\n        {\n            \"id\": \"https://api.weather.gov/alerts/urn:oid:2.49.0.1.840.0.e553a78eb2e76c08ee00c537b77b6bdc9b00773a.005.1\",\n            \"type\": \"Feature\",\n            \"geometry\": null,\n            \"properties\": {\n                \"@id\": \"https://api.weather.gov/alerts/urn:oid:2.49.0.1.840.0.e553a78eb2e76c08ee00c537b77b6bdc9b00773a.005.1\",\n                \"@type\": \"wx:Alert\",\n                \"id\": \"urn:oid:2.49.0.1.840.0.e553a78eb2e76c08ee00c537b77b6bdc9b00773a.005.1\",\n                \"areaDesc\": \"Mexico Bay NY to the St. Lawrence River\",\n                \"geocode\": {\n                    \"SAME\": [\n                        \"097045\"\n                    ],\n                    \"UGC\": [\n                        \"LOZ045\"\n                    ]\n                },\n                \"affectedZones\": [\n                    \"https://api.weather.gov/zones/forecast/LOZ045\"\n                ],\n                \"references\": [\n                    {\n                        \"@id\": \"https://api.weather.gov/alerts/urn:oid:2.49.0.1.840.0.f324634d91b7df287210abe8d836b370d8caadcc.005.1\",\n                        \"identifier\": \"urn:oid:2.49.0.1.840.0.f324634d91b7df287210abe8d836b370d8caadcc.005.1\",\n                        \"sender\": \"w-nws.webmaster@noaa.gov\",\n                        \"sent\": \"2025-12-02T15:44:00-05:00\"\n                    }\n                ],\n                \"sent\": \"2025-12-03T03:34:00-05:00\",\n                \"effective\": \"2025-12-03T03:34:00-05:00\",\n                \"onset\": \"2025-12-03T13:00:00-05:00\",\n                \"expires\": \"2025-12-03T13:00:00-05:00\",\n                \"ends\": \"2025-12-05T01:00:00-05:00\",\n                \"status\": \"Actual\",\n                \"messageType\": \"Update\",\n                \"category\": \"Met\",\n                \"severity\": \"Minor\",\n                \"certainty\": \"Likely\",\n                \"urgency\": \"Expected\",\n                \"event\": \"Small Craft Advisory\",\n                \"sender\": \"w-nws.webmaster@noaa.gov\",\n                \"senderName\": \"NWS Buffalo NY\",\n                \"headline\": \"Small Craft Advisory issued December 3 at 3:34AM EST until December 5 at 1:00AM EST by NWS Buffalo NY\",\n                \"description\": \"* WHAT...Southwest to west winds to 30 knots and waves 8 to 11\\nfeet expected.\\n\\n* WHERE...The nearshore waters of Lake Ontario from Mexico Bay\\nto the Saint Lawrence River.\\n\\n* WHEN...From 1 PM this afternoon to 1 AM EST Friday.\\n\\n* IMPACTS...Winds and/or waves will cause hazardous conditions\\nthat could capsize or damage small craft.\",\n                \"instruction\": \"Inexperienced mariners, especially those operating smaller\\nvessels, should avoid navigating in hazardous conditions.\",\n                \"response\": \"Avoid\",\n                \"parameters\": {\n                    \"AWIPSidentifier\": [\n                        \"MWWBUF\"\n                    ],\n                    \"WMOidentifier\": [\n                        \"WHUS71 KBUF 030834\"\n                    ],\n                    \"NWSheadline\": [\n                        \"SMALL CRAFT ADVISORY REMAINS IN EFFECT FROM 1 PM THIS AFTERNOON TO 1 AM EST FRIDAY\"\n                    ],\n                    \"BLOCKCHANNEL\": [\n                        \"EAS\",\n                        \"NWEM\",\n                        \"CMAS\"\n                    ],\n                    \"VTEC\": [\n                        \"/O.CON.KBUF.SC.Y.0098.251203T1800Z-251205T0600Z/\"\n                    ],\n                    \"eventEndingTime\": [\n                        \"2025-12-05T01:00:00-05:00\"\n                    ]\n                },\n                \"scope\": \"Public\",\n                \"code\": \"IPAWSv1.0\",\n                \"language\": \"en-US\",\n                \"web\": \"http://www.weather.gov\",\n                \"eventCode\": {\n                    \"SAME\": [\n                        \"NWS\"\n                    ],\n                    \"NationalWeatherService\": [\n                        \"SCY\"\n                    ]\n                }\n            }\n        },\n        {\n            \"id\": \"https://api.weather.gov/alerts/urn:oid:2.49.0.1.840.0.e553a78eb2e76c08ee00c537b77b6bdc9b00773a.004.1\",\n            \"type\": \"Feature\",\n            \"geometry\": null,\n            \"properties\": {\n                \"@id\": \"https://api.weather.gov/alerts/urn:oid:2.49.0.1.840.0.e553a78eb2e76c08ee00c537b77b6bdc9b00773a.004.1\",\n                \"@type\": \"wx:Alert\",\n                \"id\": \"urn:oid:2.49.0.1.840.0.e553a78eb2e76c08ee00c537b77b6bdc9b00773a.004.1\",\n                \"areaDesc\": \"Hamlin Beach to Sodus Bay NY; Sodus Bay to Mexico Bay NY\",\n                \"geocode\": {\n                    \"SAME\": [\n                        \"097043\",\n                        \"097044\"\n                    ],\n                    \"UGC\": [\n                        \"LOZ043\",\n                        \"LOZ044\"\n                    ]\n                },\n                \"affectedZones\": [\n                    \"https://api.weather.gov/zones/forecast/LOZ043\",\n                    \"https://api.weather.gov/zones/forecast/LOZ044\"\n                ],\n                \"references\": [\n                    {\n                        \"@id\": \"https://api.weather.gov/alerts/urn:oid:2.49.0.1.840.0.f324634d91b7df287210abe8d836b370d8caadcc.004.1\",\n                        \"identifier\": \"urn:oid:2.49.0.1.840.0.f324634d91b7df287210abe8d836b370d8caadcc.004.1\",\n                        \"sender\": \"w-nws.webmaster@noaa.gov\",\n                        \"sent\": \"2025-12-02T15:44:00-05:00\"\n                    }\n                ],\n                \"sent\": \"2025-12-03T03:34:00-05:00\",\n                \"effective\": \"2025-12-03T03:34:00-05:00\",\n                \"onset\": \"2025-12-03T19:00:00-05:00\",\n                \"expires\": \"2025-12-03T13:00:00-05:00\",\n                \"ends\": \"2025-12-05T01:00:00-05:00\",\n                \"status\": \"Actual\",\n                \"messageType\": \"Update\",\n                \"category\": \"Met\",\n                \"severity\": \"Minor\",\n                \"certainty\": \"Likely\",\n                \"urgency\": \"Expected\",\n                \"event\": \"Small Craft Advisory\",\n                \"sender\": \"w-nws.webmaster@noaa.gov\",\n                \"senderName\": \"NWS Buffalo NY\",\n                \"headline\": \"Small Craft Advisory issued December 3 at 3:34AM EST until December 5 at 1:00AM EST by NWS Buffalo NY\",\n                \"description\": \"* WHAT...Southwest to west winds to 30 knots and waves 10 to 13\\nfeet expected.\\n\\n* WHERE...The nearshore waters of Lake Ontario from Hamlin Beach\\nto Mexico Bay.\\n\\n* WHEN...From 7 PM this evening to 1 AM EST Friday.\\n\\n* IMPACTS...Winds and/or waves will cause hazardous conditions\\nthat could capsize or damage small craft.\",\n                \"instruction\": \"Inexperienced mariners, especially those operating smaller\\nvessels, should avoid navigating in hazardous conditions.\",\n                \"response\": \"Avoid\",\n                \"parameters\": {\n                    \"AWIPSidentifier\": [\n                        \"MWWBUF\"\n                    ],\n                    \"WMOidentifier\": [\n                        \"WHUS71 KBUF 030834\"\n                    ],\n                    \"NWSheadline\": [\n                        \"SMALL CRAFT ADVISORY REMAINS IN EFFECT FROM 7 PM THIS EVENING TO 1 AM EST FRIDAY\"\n                    ],\n                    \"BLOCKCHANNEL\": [\n                        \"EAS\",\n                        \"NWEM\",\n                        \"CMAS\"\n                    ],\n                    \"VTEC\": [\n                        \"/O.CON.KBUF.SC.Y.0098.251204T0000Z-251205T0600Z/\"\n                    ],\n                    \"eventEndingTime\": [\n                        \"2025-12-05T01:00:00-05:00\"\n                    ]\n                },\n                \"scope\": \"Public\",\n                \"code\": \"IPAWSv1.0\",\n                \"language\": \"en-US\",\n                \"web\": \"http://www.weather.gov\",\n                \"eventCode\": {\n                    \"SAME\": [\n                        \"NWS\"\n                    ],\n                    \"NationalWeatherService\": [\n                        \"SCY\"\n                    ]\n                }\n            }\n        },\n        {\n            \"id\": \"https://api.weather.gov/alerts/urn:oid:2.49.0.1.840.0.e553a78eb2e76c08ee00c537b77b6bdc9b00773a.002.1\",\n            \"type\": \"Feature\",\n            \"geometry\": null,\n            \"properties\": {\n                \"@id\": \"https://api.weather.gov/alerts/urn:oid:2.49.0.1.840.0.e553a78eb2e76c08ee00c537b77b6bdc9b00773a.002.1\",\n                \"@type\": \"wx:Alert\",\n                \"id\": \"urn:oid:2.49.0.1.840.0.e553a78eb2e76c08ee00c537b77b6bdc9b00773a.002.1\",\n                \"areaDesc\": \"Upper Niagara River and Buffalo Harbor; Lower Niagara River\",\n                \"geocode\": {\n                    \"SAME\": [\n                        \"096020\",\n                        \"097030\"\n                    ],\n                    \"UGC\": [\n                        \"LEZ020\",\n                        \"LOZ030\"\n                    ]\n                },\n                \"affectedZones\": [\n                    \"https://api.weather.gov/zones/forecast/LEZ020\",\n                    \"https://api.weather.gov/zones/forecast/LOZ030\"\n                ],\n                \"references\": [\n                    {\n                        \"@id\": \"https://api.weather.gov/alerts/urn:oid:2.49.0.1.840.0.f324634d91b7df287210abe8d836b370d8caadcc.002.1\",\n                        \"identifier\": \"urn:oid:2.49.0.1.840.0.f324634d91b7df287210abe8d836b370d8caadcc.002.1\",\n                        \"sender\": \"w-nws.webmaster@noaa.gov\",\n                        \"sent\": \"2025-12-02T15:44:00-05:00\"\n                    }\n                ],\n                \"sent\": \"2025-12-03T03:34:00-05:00\",\n                \"effective\": \"2025-12-03T03:34:00-05:00\",\n                \"onset\": \"2025-12-03T11:00:00-05:00\",\n                \"expires\": \"2025-12-03T13:00:00-05:00\",\n                \"ends\": \"2025-12-04T19:00:00-05:00\",\n                \"status\": \"Actual\",\n                \"messageType\": \"Update\",\n                \"category\": \"Met\",\n                \"severity\": \"Minor\",\n                \"certainty\": \"Likely\",\n                \"urgency\": \"Expected\",\n                \"event\": \"Small Craft Advisory\",\n                \"sender\": \"w-nws.webmaster@noaa.gov\",\n                \"senderName\": \"NWS Buffalo NY\",\n                \"headline\": \"Small Craft Advisory issued December 3 at 3:34AM EST until December 4 at 7:00PM EST by NWS Buffalo NY\",\n                \"description\": \"* WHAT...Southwest to west winds 15 to 20 knots expected.\\n\\n* WHERE...The Niagara River and Buffalo Harbor.\\n\\n* WHEN...From 11 AM this morning to 7 PM EST Thursday.\\n\\n* IMPACTS...Winds and/or waves will cause hazardous conditions\\nthat could capsize or damage small craft.\",\n                \"instruction\": \"Inexperienced mariners, especially those operating smaller\\nvessels, should avoid navigating in hazardous conditions.\",\n                \"response\": \"Avoid\",\n                \"parameters\": {\n                    \"AWIPSidentifier\": [\n                        \"MWWBUF\"\n                    ],\n                    \"WMOidentifier\": [\n                        \"WHUS71 KBUF 030834\"\n                    ],\n                    \"NWSheadline\": [\n                        \"SMALL CRAFT ADVISORY REMAINS IN EFFECT FROM 11 AM THIS MORNING TO 7 PM EST THURSDAY\"\n                    ],\n                    \"BLOCKCHANNEL\": [\n                        \"EAS\",\n                        \"NWEM\",\n                        \"CMAS\"\n                    ],\n                    \"VTEC\": [\n                        \"/O.CON.KBUF.SC.Y.0098.251203T1600Z-251205T0000Z/\"\n                    ],\n                    \"eventEndingTime\": [\n                        \"2025-12-04T19:00:00-05:00\"\n                    ]\n                },\n                \"scope\": \"Public\",\n                \"code\": \"IPAWSv1.0\",\n                \"language\": \"en-US\",\n                \"web\": \"http://www.weather.gov\",\n                \"eventCode\": {\n                    \"SAME\": [\n                        \"NWS\"\n                    ],\n                    \"NationalWeatherService\": [\n                        \"SCY\"\n                    ]\n                }\n            }\n        },\n        {\n            \"id\": \"https://api.weather.gov/alerts/urn:oid:2.49.0.1.840.0.e553a78eb2e76c08ee00c537b77b6bdc9b00773a.003.1\",\n            \"type\": \"Feature\",\n            \"geometry\": null,\n            \"properties\": {\n                \"@id\": \"https://api.weather.gov/alerts/urn:oid:2.49.0.1.840.0.e553a78eb2e76c08ee00c537b77b6bdc9b00773a.003.1\",\n                \"@type\": \"wx:Alert\",\n                \"id\": \"urn:oid:2.49.0.1.840.0.e553a78eb2e76c08ee00c537b77b6bdc9b00773a.003.1\",\n                \"areaDesc\": \"Niagara River to Hamlin Beach NY\",\n                \"geocode\": {\n                    \"SAME\": [\n                        \"097042\"\n                    ],\n                    \"UGC\": [\n                        \"LOZ042\"\n                    ]\n                },\n                \"affectedZones\": [\n                    \"https://api.weather.gov/zones/forecast/LOZ042\"\n                ],\n                \"references\": [\n                    {\n                        \"@id\": \"https://api.weather.gov/alerts/urn:oid:2.49.0.1.840.0.f324634d91b7df287210abe8d836b370d8caadcc.003.1\",\n                        \"identifier\": \"urn:oid:2.49.0.1.840.0.f324634d91b7df287210abe8d836b370d8caadcc.003.1\",\n                        \"sender\": \"w-nws.webmaster@noaa.gov\",\n                        \"sent\": \"2025-12-02T15:44:00-05:00\"\n                    }\n                ],\n                \"sent\": \"2025-12-03T03:34:00-05:00\",\n                \"effective\": \"2025-12-03T03:34:00-05:00\",\n                \"onset\": \"2025-12-03T11:00:00-05:00\",\n                \"expires\": \"2025-12-03T13:00:00-05:00\",\n                \"ends\": \"2025-12-04T22:00:00-05:00\",\n                \"status\": \"Actual\",\n                \"messageType\": \"Update\",\n                \"category\": \"Met\",\n                \"severity\": \"Minor\",\n                \"certainty\": \"Likely\",\n                \"urgency\": \"Expected\",\n                \"event\": \"Small Craft Advisory\",\n                \"sender\": \"w-nws.webmaster@noaa.gov\",\n                \"senderName\": \"NWS Buffalo NY\",\n                \"headline\": \"Small Craft Advisory issued December 3 at 3:34AM EST until December 4 at 10:00PM EST by NWS Buffalo NY\",\n                \"description\": \"* WHAT...Southwest to west winds to 30 knots and waves 7 to 10\\nfeet expected.\\n\\n* WHERE...The nearshore waters of Lake Ontario from the Niagara\\nRiver to Hamlin Beach.\\n\\n* WHEN...From 11 AM this morning to 10 PM EST Thursday.\\n\\n* IMPACTS...Winds and/or waves will cause hazardous conditions\\nthat could capsize or damage small craft.\",\n                \"instruction\": \"Inexperienced mariners, especially those operating smaller\\nvessels, should avoid navigating in hazardous conditions.\",\n                \"response\": \"Avoid\",\n                \"parameters\": {\n                    \"AWIPSidentifier\": [\n                        \"MWWBUF\"\n                    ],\n                    \"WMOidentifier\": [\n                        \"WHUS71 KBUF 030834\"\n                    ],\n                    \"NWSheadline\": [\n                        \"SMALL CRAFT ADVISORY REMAINS IN EFFECT FROM 11 AM THIS MORNING TO 10 PM EST THURSDAY\"\n                    ],\n                    \"BLOCKCHANNEL\": [\n                        \"EAS\",\n                        \"NWEM\",\n                        \"CMAS\"\n                    ],\n                    \"VTEC\": [\n                        \"/O.CON.KBUF.SC.Y.0098.251203T1600Z-251205T0300Z/\"\n                    ],\n                    \"eventEndingTime\": [\n                        \"2025-12-04T22:00:00-05:00\"\n                    ]\n                },\n                \"scope\": \"Public\",\n                \"code\": \"IPAWSv1.0\",\n                \"language\": \"en-US\",\n                \"web\": \"http://www.weather.gov\",\n                \"eventCode\": {\n                    \"SAME\": [\n                        \"NWS\"\n                    ],\n                    \"NationalWeatherService\": [\n                        \"SCY\"\n                    ]\n                }\n            }\n        },\n        {\n            \"id\": \"https://api.weather.gov/alerts/urn:oid:2.49.0.1.840.0.e553a78eb2e76c08ee00c537b77b6bdc9b00773a.001.1\",\n            \"type\": \"Feature\",\n            \"geometry\": null,\n            \"properties\": {\n                \"@id\": \"https://api.weather.gov/alerts/urn:oid:2.49.0.1.840.0.e553a78eb2e76c08ee00c537b77b6bdc9b00773a.001.1\",\n                \"@type\": \"wx:Alert\",\n                \"id\": \"urn:oid:2.49.0.1.840.0.e553a78eb2e76c08ee00c537b77b6bdc9b00773a.001.1\",\n                \"areaDesc\": \"Ripley to Dunkirk NY; Dunkirk to Buffalo NY\",\n                \"geocode\": {\n                    \"SAME\": [\n                        \"096040\",\n                        \"096041\"\n                    ],\n                    \"UGC\": [\n                        \"LEZ040\",\n                        \"LEZ041\"\n                    ]\n                },\n                \"affectedZones\": [\n                    \"https://api.weather.gov/zones/forecast/LEZ040\",\n                    \"https://api.weather.gov/zones/forecast/LEZ041\"\n                ],\n                \"references\": [\n                    {\n                        \"@id\": \"https://api.weather.gov/alerts/urn:oid:2.49.0.1.840.0.f324634d91b7df287210abe8d836b370d8caadcc.001.1\",\n                        \"identifier\": \"urn:oid:2.49.0.1.840.0.f324634d91b7df287210abe8d836b370d8caadcc.001.1\",\n                        \"sender\": \"w-nws.webmaster@noaa.gov\",\n                        \"sent\": \"2025-12-02T15:44:00-05:00\"\n                    }\n                ],\n                \"sent\": \"2025-12-03T03:34:00-05:00\",\n                \"effective\": \"2025-12-03T03:34:00-05:00\",\n                \"onset\": \"2025-12-03T07:00:00-05:00\",\n                \"expires\": \"2025-12-03T13:00:00-05:00\",\n                \"ends\": \"2025-12-04T22:00:00-05:00\",\n                \"status\": \"Actual\",\n                \"messageType\": \"Update\",\n                \"category\": \"Met\",\n                \"severity\": \"Minor\",\n                \"certainty\": \"Likely\",\n                \"urgency\": \"Expected\",\n                \"event\": \"Small Craft Advisory\",\n                \"sender\": \"w-nws.webmaster@noaa.gov\",\n                \"senderName\": \"NWS Buffalo NY\",\n                \"headline\": \"Small Craft Advisory issued December 3 at 3:34AM EST until December 4 at 10:00PM EST by NWS Buffalo NY\",\n                \"description\": \"* WHAT...Southwest to west winds to 30 knots and waves 7 to 10\\nfeet expected.\\n\\n* WHERE...The nearshore waters of Lake Erie from Ripley to\\nBuffalo.\\n\\n* WHEN...From 7 AM this morning to 10 PM EST Thursday.\\n\\n* IMPACTS...Winds and/or waves will cause hazardous conditions\\nthat could capsize or damage small craft.\",\n                \"instruction\": \"Inexperienced mariners, especially those operating smaller\\nvessels, should avoid navigating in hazardous conditions.\",\n                \"response\": \"Avoid\",\n                \"parameters\": {\n                    \"AWIPSidentifier\": [\n                        \"MWWBUF\"\n                    ],\n                    \"WMOidentifier\": [\n                        \"WHUS71 KBUF 030834\"\n                    ],\n                    \"NWSheadline\": [\n                        \"SMALL CRAFT ADVISORY REMAINS IN EFFECT FROM 7 AM THIS MORNING TO 10 PM EST THURSDAY\"\n                    ],\n                    \"BLOCKCHANNEL\": [\n                        \"EAS\",\n                        \"NWEM\",\n           
